vi "I2C Initialize.vi"(8 "error in (no error)":errorcluster, 11 "I2C Task In":T1) -> (0 "error out":errorcluster, 3 "I2C Task Out":T1)   [LabVIEW 2017, in "I2C.lvlib"]
doc: "Initializes the I2C communication."
uses:
  <vilib>/robotics/Protocols/I2C/DAQmx/I2C.lvlib
  <vilib>/robotics/Protocols/I2C/DAQmx/Private/I2C Tasks.ctl
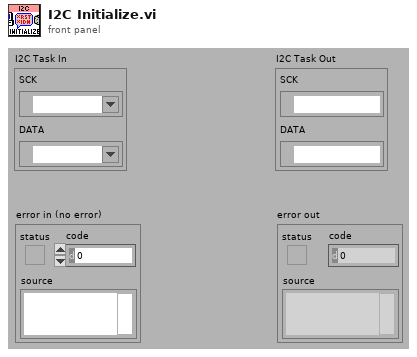
[diagram p1: front panel]
types:
  T1 = typedef "I2C.lvlib/I2C Tasks.ctl" = cluster{"SCK":refnum<k21>, "DATA":refnum<k21>}
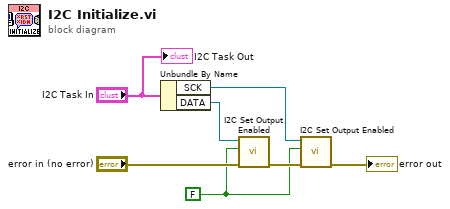
[diagram p0: block diagram]
diagram:
  w4 = FALSE ("Output Enabled (T:Enable)")
  n1 = Unbundle By Name("I2C Task In") -> ("SCK"=w2:refnum<k21>, "DATA"=w3:refnum<k21>)
  n2 = call <vilib>:"I2C Set Output Enabled.vi"("error in (no error)"="error in (no error)", "Output Enabled (T:Enable)"=w4, "Task In"=w3) -> ("error out"=w5:errorcluster)  [unwired: 7 in, 1 out]
  n3 = call <vilib>:"I2C Set Output Enabled.vi"("error in (no error)"=w5, "Output Enabled (T:Enable)"=w4, "Task In"=w2) -> ("error out"=→"error out":errorcluster)  [unwired: 7 in, 1 out]
  "I2C Task Out" <- "I2C Task In"
